vi "Get Sys (To) Period.vi"(8 "error in (no error)":errorcluster, 11 "VISA resource name":refnum<visa-resource-name>) -> (0 "error out":errorcluster, 2 "Period":dbl, 3 "VISA resource name out":refnum<visa-resource-name>)   [LabVIEW 2012, in "Quantum Composers 9000 Series.lvlib"]
doc: "This VI is used to read the base timer (i.e. System (To)) period.\n\nValid Range: 2.0E-7 to 5000 sec"
uses:
  Quantum Composers 9000 Series.lvlib
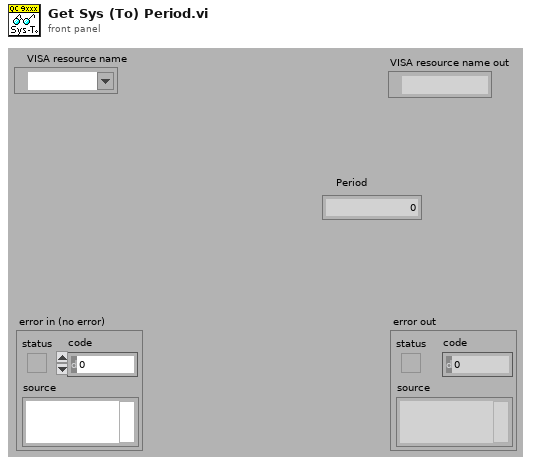
[diagram p1: front panel]
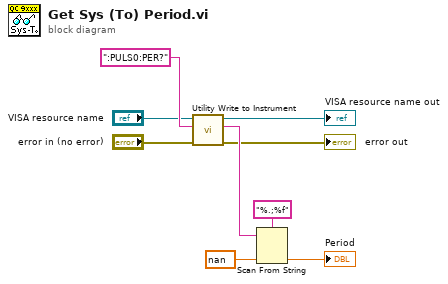
[diagram p0: block diagram]
diagram:
  n1 = call "Utility Write to Instrument.vi"("error in (no error)"="error in (no error)", "Write Buffer"=":PULS0:PER?", "VISA resource name"="VISA resource name") -> ("error out"=→"error out":errorcluster, "Read Buffer"=w9:string, "VISA resource name out"=→"VISA resource name out":refnum<visa-resource-name>)  [unwired: 6 out]
  n2 = Scan From String(format string="%.;%f", input string=w9, default 1=nan ("default value 1")) -> (output 1=→"Period":dbl)  [unwired: 2 in, 3 out]
